vi "Vision Processing.vi"(8 "error in (no error)":errorcluster, 11 "Boolean":bool=TRUE) -> (3 "Distances":T5(array[cluster]))   [LabVIEW 2013]
doc: "This VI runs in parallel to other tasks. It gets images from the camera, processes them for color or shape and use that information to affect robot behavior."
uses:
  <vilib>/Rock Robotics/WPI/Camera/WPI_CameraImageSize.ctl
  Program Files (x86)/National Instruments/LabVIEW 2013/examples/FRC/Vision/2014 Target Detection/TargetType.ctl
  <vilib>/Rock Robotics/WPI/Camera/WPI_CameraWhite Balance Values.ctl
  <vilib>/Rock Robotics/WPI/Camera/WPI_CameraExposure Values.ctl
  <vilib>/Rock Robotics/WPI/Camera/WPI_CameraFrameRate.ctl
panel:
  out "Image":T1(plugin-control)
  out "Mask":T1(plugin-control)
  in  "Area Size Limit %":dbl=0.06 format="%#_13g"
  in  "Score Cutoff":dbl(slide)=54.248366013071895 scale=0.0..100.0
  out "Target Info":T3(array[cluster])
  in  "Camera Type":enum16{"206", "1011", "1013"}(ring)=enum."1011"
  in  "Color Components":T4={"Hue"={112.0, 144.0}, "Sat"={198.0, 255.0}, "Val"={231.0, 255.0}} {"Val" scale=0.0..255.0; "Sat" scale=0.0..255.0; "Hue" scale=0.0..255.0 scale format="%#_3g"}
  in  "Std Devs":cluster{"Hue":dbl, "Sat":dbl, "Val":dbl}={"Hue"=4.0, "Sat"=6.0, "Val"=4.0}
  in  "Image Size":T6=enum."320x240"
  out "resulting string":string="10.34.92.11"
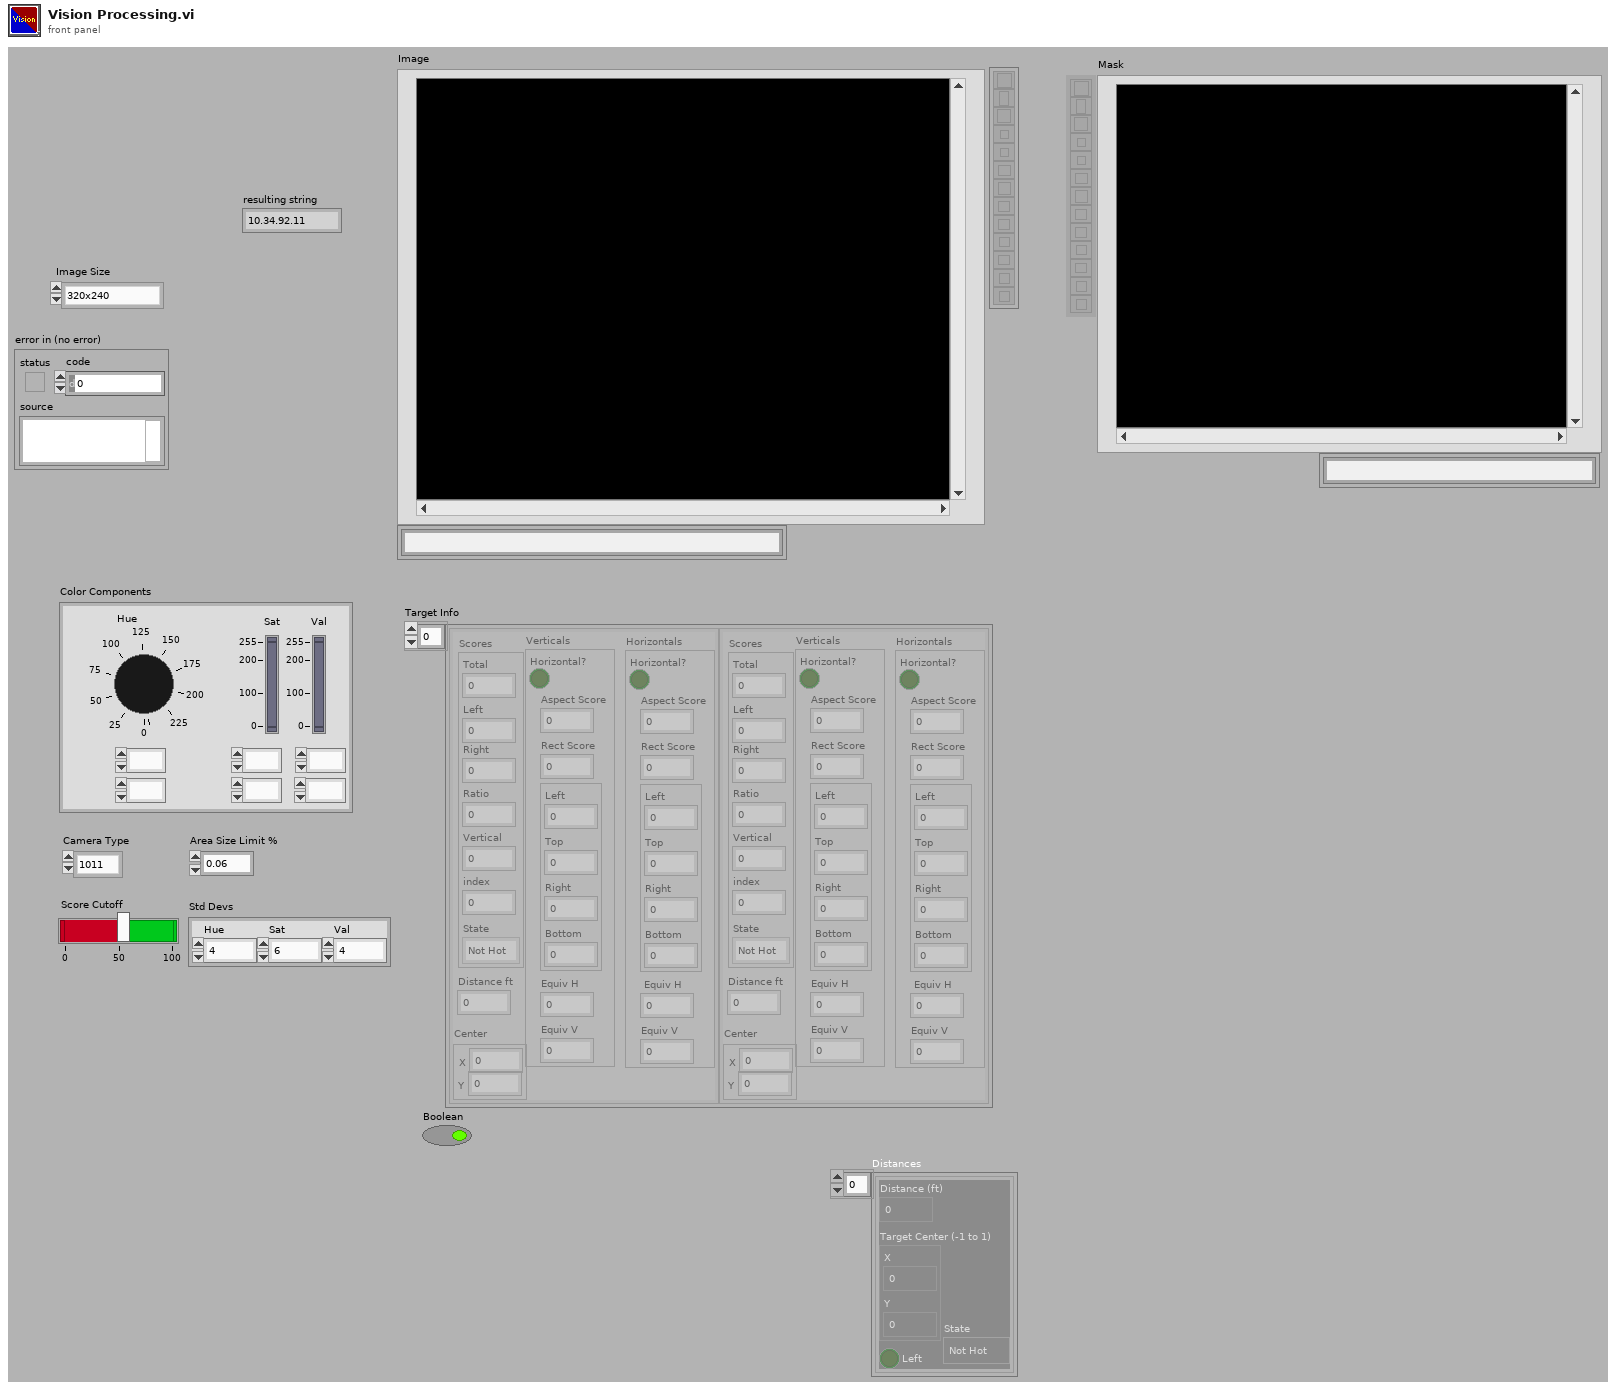
[diagram p1: front panel]
types:
  T1 = typedef "IMAQ Image.ctl" = refnum<image>
  T2 = typedef "TargetType.ctl" = enum16{"Not Hot", "Hot"}
  T3 = cluster{"Scores":cluster{"Total":dbl, "Left":dbl, "Right":dbl, "Ratio":dbl, "Vertical":dbl, "index":i32, "State":T2}, "Verticals":cluster{"Horizontal?":bool, "Aspect Score":dbl, "Rect Score":dbl, cluster{"Left":dbl, "Top":dbl, "Right":dbl, "Bottom":dbl}, "Equiv H":dbl, "Equiv V":dbl}, "Horizontals":cluster{"Horizontal?":bool, "Aspect Score":dbl, "Rect Score":dbl, cluster{"Left":dbl, "Top":dbl, "Right":dbl, "Bottom":dbl}, "Equiv H":dbl, "Equiv V":dbl}, "Distance ft":dbl, "Center":cluster{"X":dbl, "Y":dbl}}[]
  T4 = cluster{"Hue":cluster{dbl, dbl}, "Sat":cluster{dbl, dbl}, "Val":cluster{dbl, dbl}}
  T5 = cluster{"Distance (ft)":dbl, "Target Center (-1 to 1)":cluster{"X":dbl, "Y":dbl}, "Left":bool, "State":T2}[]
  T6 = typedef "WPI_CameraImageSize.ctl" = enum16{"640x480", "320x240", "160x120"}
  T7 = typedef "WPI_CameraFrameRate.ctl" = u32
  T8 = typedef "WPI_CameraExposure Values.ctl" = enum16{"Auto", "Flicker-free 50 Hz", "Flicker-free 60 Hz", "Hold current"}
  T9 = typedef "WPI_CameraWhite Balance Values.ctl" = enum16{"Auto", "Fixed indoor", "Fixed outdoor 1", "Fixed outdoor 2", "Fixed fluorescent 1", "Fixed fluorescent 2", "Hold current"}
  T10 = typedef "WPI_CameraDevRef.ctl" = cluster{"Camera Address":string, "CameraStatus":errorcluster, "Acquire Image Notifier":refnum<notifier>}
  T11 = typedef "Image Type" = u32
  T12 = cluster{"Horizontal":bool, "Aspect Score":dbl, "Rect Score":dbl, cluster{"Left":dbl, "Top":dbl, "Right":dbl, "Bottom":dbl}, "Equiv H":dbl, "Equiv V":dbl}[]
  T13 = cluster{cluster{dbl, dbl}, cluster{dbl, dbl}, cluster{dbl, dbl}}
  T14 = cluster{"Scores":cluster{"Total":dbl, "Left":dbl, "Right":dbl, "Ratio":dbl, "Vertical":dbl, "index":i32, "State":T2}, "Verticals":cluster{"Horizontal?":bool, "Aspect Score":dbl, "Rect Score":dbl, cluster{"Left":dbl, "Top":dbl, "Right":dbl, "Bottom":dbl}, "Equiv H":dbl, "Equiv V":dbl}, "Horizontals":cluster{"Horizontal?":bool, "Aspect Score":dbl, "Rect Score":dbl, cluster{"Left":dbl, "Top":dbl, "Right":dbl, "Bottom":dbl}, "Equiv H":dbl, "Equiv V":dbl}, "Validated":bool}[]
  T15 = cluster{"Scores":cluster{"Total":dbl, "Left":dbl, "Right":dbl, "Ratio":dbl, "Vertical":dbl, "index":i32, "State":T2}, "Verticals":cluster{"Horizontal?":bool, "Aspect Score":dbl, "Rect Score":dbl, cluster{"Left":dbl, "Top":dbl, "Right":dbl, "Bottom":dbl}, "Equiv H":dbl, "Equiv V":dbl}, "Horizontals":cluster{"Horizontal?":bool, "Aspect Score":dbl, "Rect Score":dbl, cluster{"Left":dbl, "Top":dbl, "Right":dbl, "Bottom":dbl}, "Equiv H":dbl, "Equiv V":dbl}, "Distance (ft)":dbl, "Target Center (-1 to 1)":cluster{"X":dbl, "Y":dbl}}[]
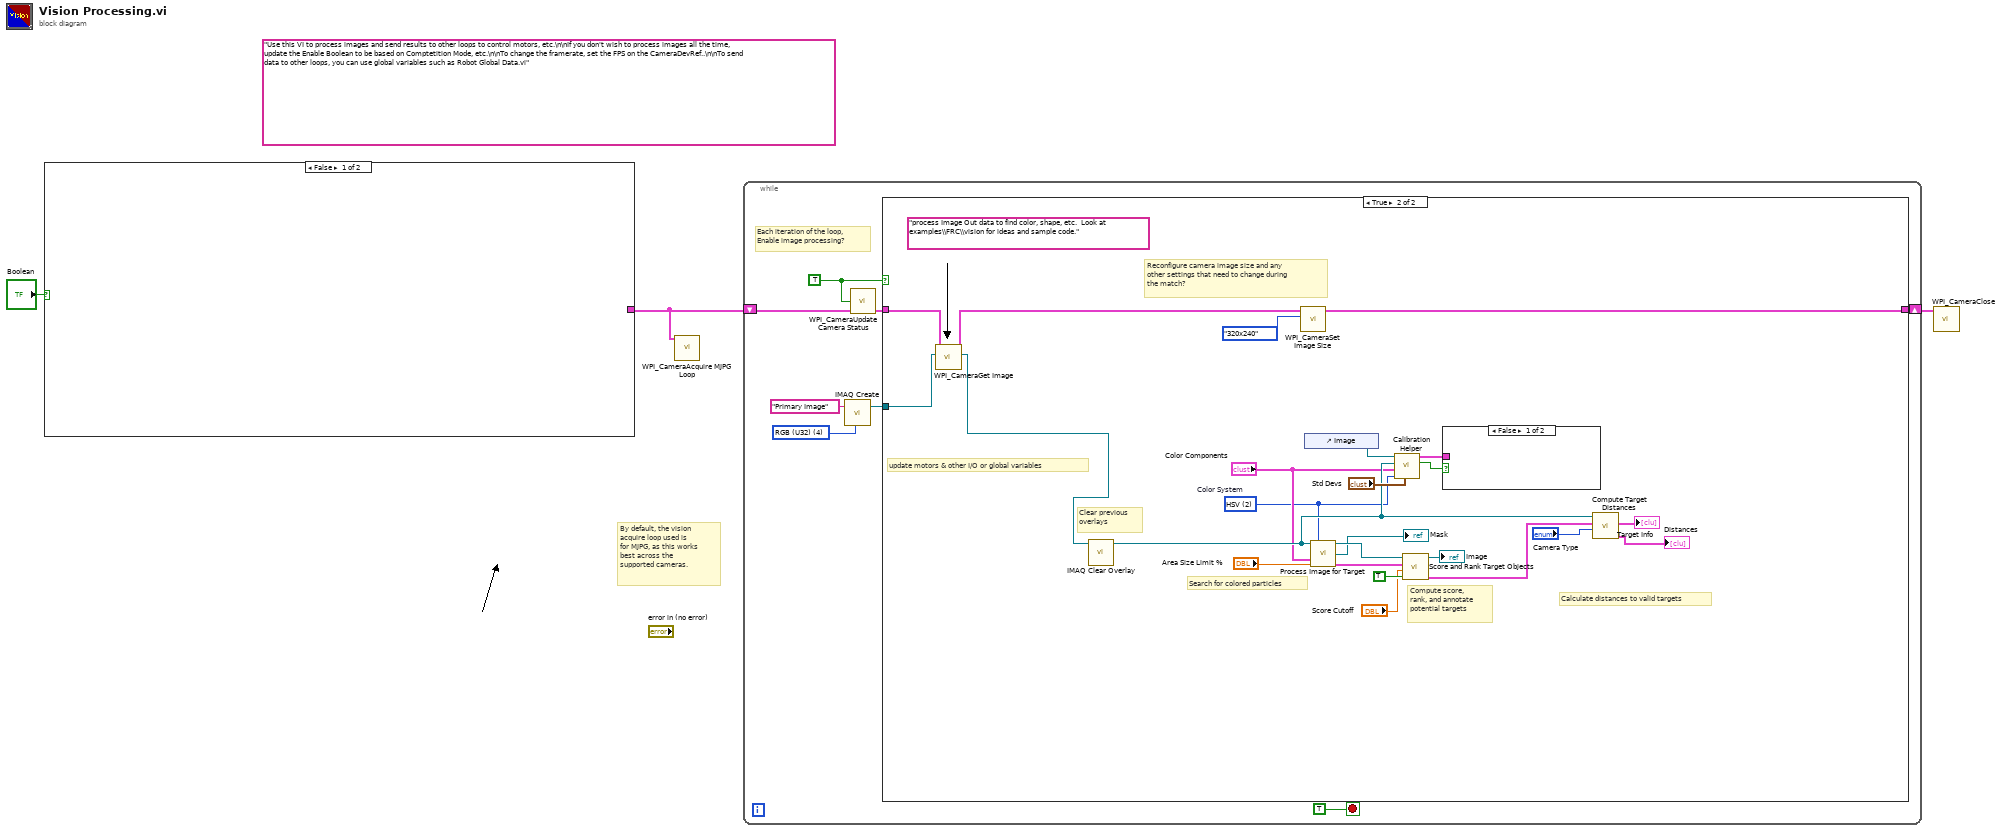
[diagram p0: block diagram]
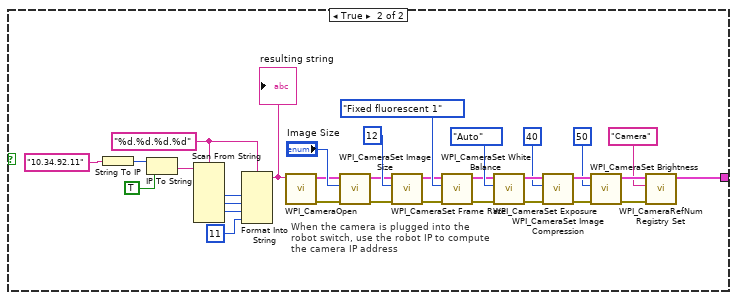
[diagram p2: hidden frame]
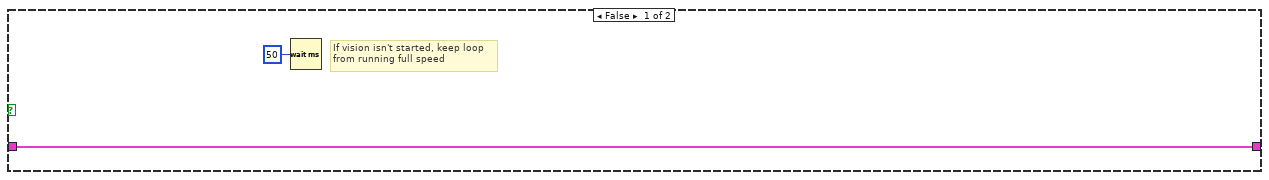
[diagram p3: hidden frame]
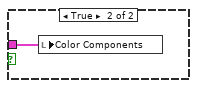
[diagram p4: hidden frame]
diagram:
  (unwired) "Use this VI to process images and send results to other loops to control motors, etc.\n\nIf you don't wish to process images all the time, update the Enable Boolean to be based on Comptetition Mode, etc.\n\nTo change the framerate, set the FPS on the CameraDevRef..\n\nTo send data to other loops, you can use global variables such as Robot Global Data.vi"
  # "By default, the vision\nacquire loop used is\nfor MJPG, as this works\nbest across the\nsupported cameras."
  n1 = case shown="False" "Boolean" {
    tunnel: [_ w35] -> w2
    frame False {
    }
    frame True {
      w31 = "%d.%d.%d.%d" ("format string")
      # "When the camera is plugged into the\nrobot switch, use the robot IP to compute\nthe camera IP address"
      n2 = String To IP(1:"10.34.92.11" ("name")) -> (0:w24:u32)
      n3 = IP To String(1:TRUE ("dot notation? (F)"), 2:w24) -> (0:w26:string)
      n4 = Scan From String(format string=w31, input string=w26) -> (output 1=w27:i32, output 2=w28:i32, output 3=w29:i32)  [unwired: 7 in, 3 out]
      n5 = Format Into String(format string=w31, w27, w28, w29, 11 ("Compression")) -> (resulting string=w34:string)  [unwired: 2 in, 1 out]
      "resulting string" <- w34
      n6 = call <vilib>:"WPI_CameraOpen.vi"("Camera Address"=w34) -> ("error out"=w13:errorcluster, "CameraDevRef"=w12:T10)  [unwired: 1 in, 8 out]
      n7 = call <vilib>:"WPI_CameraSet Image Size.vi"("error in (no error)"=w13, "Image Size"="Image Size", "CameraDevRef"=w12) -> ("error out"=w14:errorcluster, "CameraDevRef Out"=w11:T10)  [unwired: 7 out]
      n8 = call <vilib>:"WPI_CameraSet Frame Rate.vi"("error in (no error)"=w14, "Frame Rate (fps)"=T7 12, "CameraDevRef"=w11) -> ("error out"=w15:errorcluster, "CameraDevRef Out"=w9:T10)  [unwired: 7 out]
      n9 = call <vilib>:"WPI_CameraSet White Balance.vi"("error in (no error)"=w15, "White Balance"=WPI_CameraWhite_Balance_Values."Fixed fluorescent 1", "CameraDevRef"=w9) -> ("error out"=w16:errorcluster, "CameraDevRef Out"=w10:T10)  [unwired: 7 out]
      n10 = call <vilib>:"WPI_CameraSet Exposure.vi"("error in (no error)"=w16, "Exposure"=WPI_CameraExposure_Values."Auto", "CameraDevRef"=w10) -> ("error out"=w17:errorcluster, "CameraDevRef Out"=w7:T10)  [unwired: 7 out]
      n11 = call <vilib>:"WPI_CameraSet Image Compression.vi"("error in (no error)"=w17, "Compression"=40, "CameraDevRef"=w7) -> ("error out"=w18:errorcluster, "CameraDevRef Out"=w8:T10)  [unwired: 7 out]
      n12 = call <vilib>:"WPI_CameraSet Brightness.vi"("error in (no error)"=w18, "Brightness"=50, "CameraDevRef"=w8) -> ("error out"=w20:errorcluster, "CameraDevRef Out"=w19:T10)  [unwired: 7 out]
      n13 = call <vilib>:"WPI_CameraRefNum Registry Set.vi"("error in (no error)"=w20, "refnum name"="Camera", "CameraDevRef"=w19) -> ("CameraDevRef"=w35:T10)  [unwired: 8 out]
    }
  }
  n14 = call <vilib>:"WPI_CameraAcquire MJPG Loop.vi"("CameraDevRef"=w2) -> ()  [unwired: 11 in]
  n15 = while {
    shift-right: [w42] -> w3
    shift-left: w2 -> [w36]
    stop <- TRUE stop-if-true
    w39 = T11 4 items=["Grayscale (U8)", "Grayscale (I16)", "Grayscale (SGL)", "Complex (CSG)", "RGB (U32)", "HSL (U32)", "RGB (U64)"] ("Image Type")
    w40 = TRUE
    # "Each iteration of the loop,\nEnable image processing?"
    n16 = call "IMAQ Create"("Image Name"="Primary Image", "Image Type"=w39) -> ("New Image"=w37:T1)  [unwired: 2 in, 2 out]
    n17 = call <vilib>:"WPI_CameraUpdate Camera Status.vi"("CameraDevRef In"=w36, "Enable Vision"=w40) -> ("CameraDevRef Out"=w41:T10)  [unwired: 3 in]
    n18 = case shown="True" w40 {
      tunnel: [w45 w69] -> w42
      tunnel: w41 -> [w45 w68]
      tunnel: w37 -> [_ w46]
      frame False {
        # "If vision isn't started, keep loop\nfrom running full speed"
        n19 = Wait (ms)(milliseconds to wait=u32 50) -> ()  [unwired: 1 out]
      }
      frame True {
        w58 = u16 2 items=["RGB", "HSL", "HSV", "HSI"]  # Color System
        (unwired) "process Image Out data to find color, shape, etc.  Look at examples\\FRC\\vision for ideas and sample code."
        # "Clear previous\noverlays"
        # "Calculate distances to valid targets"
        # "Search for colored particles"
        # "Compute score,\nrank, and annotate\npotential targets"
        # "update motors & other I/O or global variables"
        # "Reconfigure camera image size and any\nother settings that need to change during\nthe match?"
        n20 = call <vilib>:"WPI_CameraGet Image.vi"("Image"=w46, "CameraDevRef"=w68) -> ("Image Out"=w48:T1, "CameraDevRef Out"=w67:T10)  [unwired: 1 in, 7 out]
        n21 = call "IMAQ Clear Overlay"("Image"=w48) -> ("Image Out"=w60:T1)  [unwired: 9 in, 1 out]
        n22 = call <vilib>:"WPI_CameraSet Image Size.vi"("Image Size"=WPI_CameraImageSize."320x240", "CameraDevRef"=w67) -> ("CameraDevRef Out"=w69:T10)  [unwired: 1 in, 8 out]
        n23 = control-ref of="Image"() -> (w62:refnum<vi>)
        n24 = call "Process Image for Target.vi"("Src Image"=w60, "Color Mode"=w58, "Color Components"="Color Components", "Area Cutoff %"="Area Size Limit %") -> ("Src Image Out"=w51:T1, "Threshold"=→"Mask":T1, "Particles"=w54:T12)  [unwired: 9 in]
        n25 = call "Calibration Helper.vi"("Std Devs"="Std Devs", "Color Mode"=w58, "Color Components"="Color Components", "Image"=w60, "Image Ctl Refnum"=w62) -> ("Changed"=w65:bool, "output color"=w64:T13)  [unwired: 5 in]
        n26 = call "Score and Rank Target Objects.vi"("Annotate"=TRUE, "Score Limit"="Score Cutoff", "Particles"=w54, "Image in"=w51) -> ("Target Info"=w55:T14, "Annotated Image"=→"Image":T1)  [unwired: 6 in]
        n27 = case shown="False" w65 {
          tunnel: w64 -> [_ w70]
          frame False {
          }
          frame True {
            n28 = local write "Color Components"(w70) -> ()
          }
        }
        n29 = call "Compute Target Distances.vi"("Camera Type"="Camera Type", "Target Info"=w55, "Image in"=w60) -> ("Distances"=→"Distances":T5, "Target Info"=→"Target Info":T15)  [unwired: 6 in, 1 out]
      }
    }
  }
  n30 = call <vilib>:"WPI_CameraClose.vi"("CameraDevRef"=w3) -> ()  [unwired: 1 in, 10 out]
